vi "Global pulses.vi"() -> ()   [LabVIEW 2017]
panel:
  out "global y reached":bool
  out "global x reached":bool
  in  "speed level":T1(ring)
  out "y":dbl
  out "x":dbl
  out "Top pressed":dbl
  out "time not moving":dbl
  out "Frequency M2":dbl
  out "Frequncy M1":dbl
  out "Frequency":dbl
  out "Time variable":dbl
  out "Enc M2":dbl
  out "Enc M1":dbl
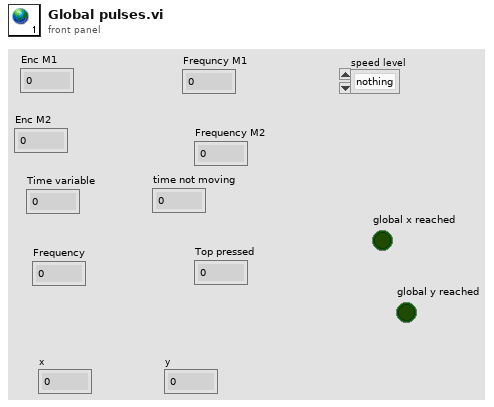
[diagram p1: front panel]
types:
  T1 = enum16{"nothing", "high speed", "medium speed", "low speed"}
diagram:
